vi "SIMPLE_Bulk_Stat.vi"() -> ()   [LabVIEW 2016]
uses:
  <vilib>/Instr/_visa.llb/VISA Set IO Buffer Mask.ctl
  <vilib>/Utility/miscctls.llb/LVPointTypeDef.ctl
  REV_2.lvlib
  <vilib>/Instr/_visa.llb/VISA Configure Serial Port (Instr).vi
  REV2_Stat_Addr.ctl
panel:
  out "Waveform Chart":dbl(graph)=240.78979051288226
  in  "Enum":enum16{"One_by_One", "Bulk"}(ring)
  in  "Stat_to_Read":T1[](array[typedef])=[8, 9] items=["Torque Enable", "Homing Complete", "Goal Id", "Goal Iq", "Goal Velo", "Goal Posi", "Present Id", "Present Iq", "Present Velo", "Present Posi", "Bus Voltage", "Temperature Winding", "Temperature MOSFET", "Temperature IC", "Error Status", "Iq_Temps"]
  in  "Data_to_Write":dbl[][](array[numeric])=[[0.0], [0.0], [0.0], [0.0], [0.0], [0.0], [0.0], [0.0], [0.0], [0.0], [0.0], [0.0]]
  in  "Stat_to_Write":T1[](array[typedef])=[3] items=["Torque Enable", "Homing Complete", "Goal Id", "Goal Iq", "Goal Velo", "Goal Posi", "Present Id", "Present Iq", "Present Velo", "Present Posi", "Bus Voltage", "Temperature Winding", "Temperature MOSFET", "Temperature IC", "Error Status", "Iq_Temps"]
  in  "IDs":u8[](array[numeric])=[1, 2, 3, 4, 5, 6, 7, 8, 9, 10, 11, 12]
  out "Data_2D":dbl[][](array[numeric])=[[-0.09640240669250488, 7372.0263671875], [-1.2603185176849365, -5385.19287109375], [-0.42314088344573975, 130929.453125], [-0.14840322732925415, 13840.2578125], [-0.6294983625411987, -4865.42578125], [0.10544928908348083, 128472.46875], [-1.5680679082870483, 28076.017578125], [-0.011024624109268188, -5347.7939453125], [1.180788278579712, 128403.328125], [-0.07580620050430298, 30035.9765625], [-0.3092707395553589, -5952.68359375], [-0.6351131200790405, 130700.546875]]
  in  "R/W":bool
  in  "Baud rate":u32=8000000
  in  "Com port":refnum<visa-resource-name>="COM7"
  in  "stop":bool
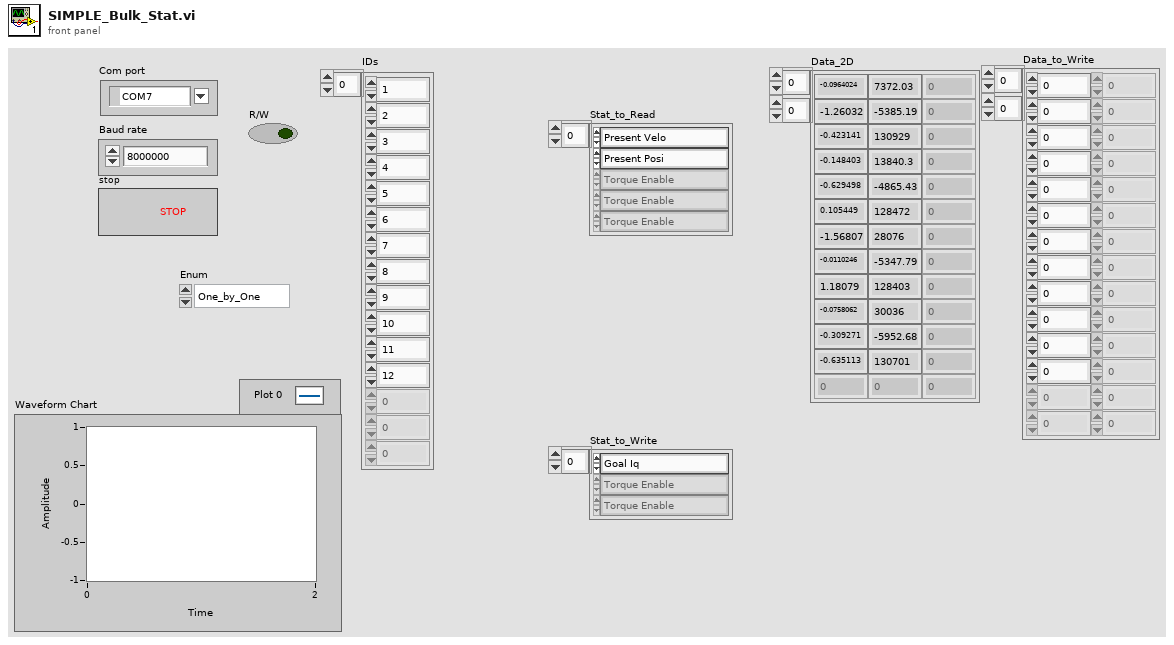
[diagram p1: front panel]
types:
  T1 = typedef "REV_2.lvlib/REV2_Stat_Addr.ctl" = u8
  T2 = typedef "LVPointTypeDef.ctl" = cluster{"Horizontal":i16, "Vertical":i16}
  T3 = typedef "VISA Set IO Buffer Mask.ctl" = u16
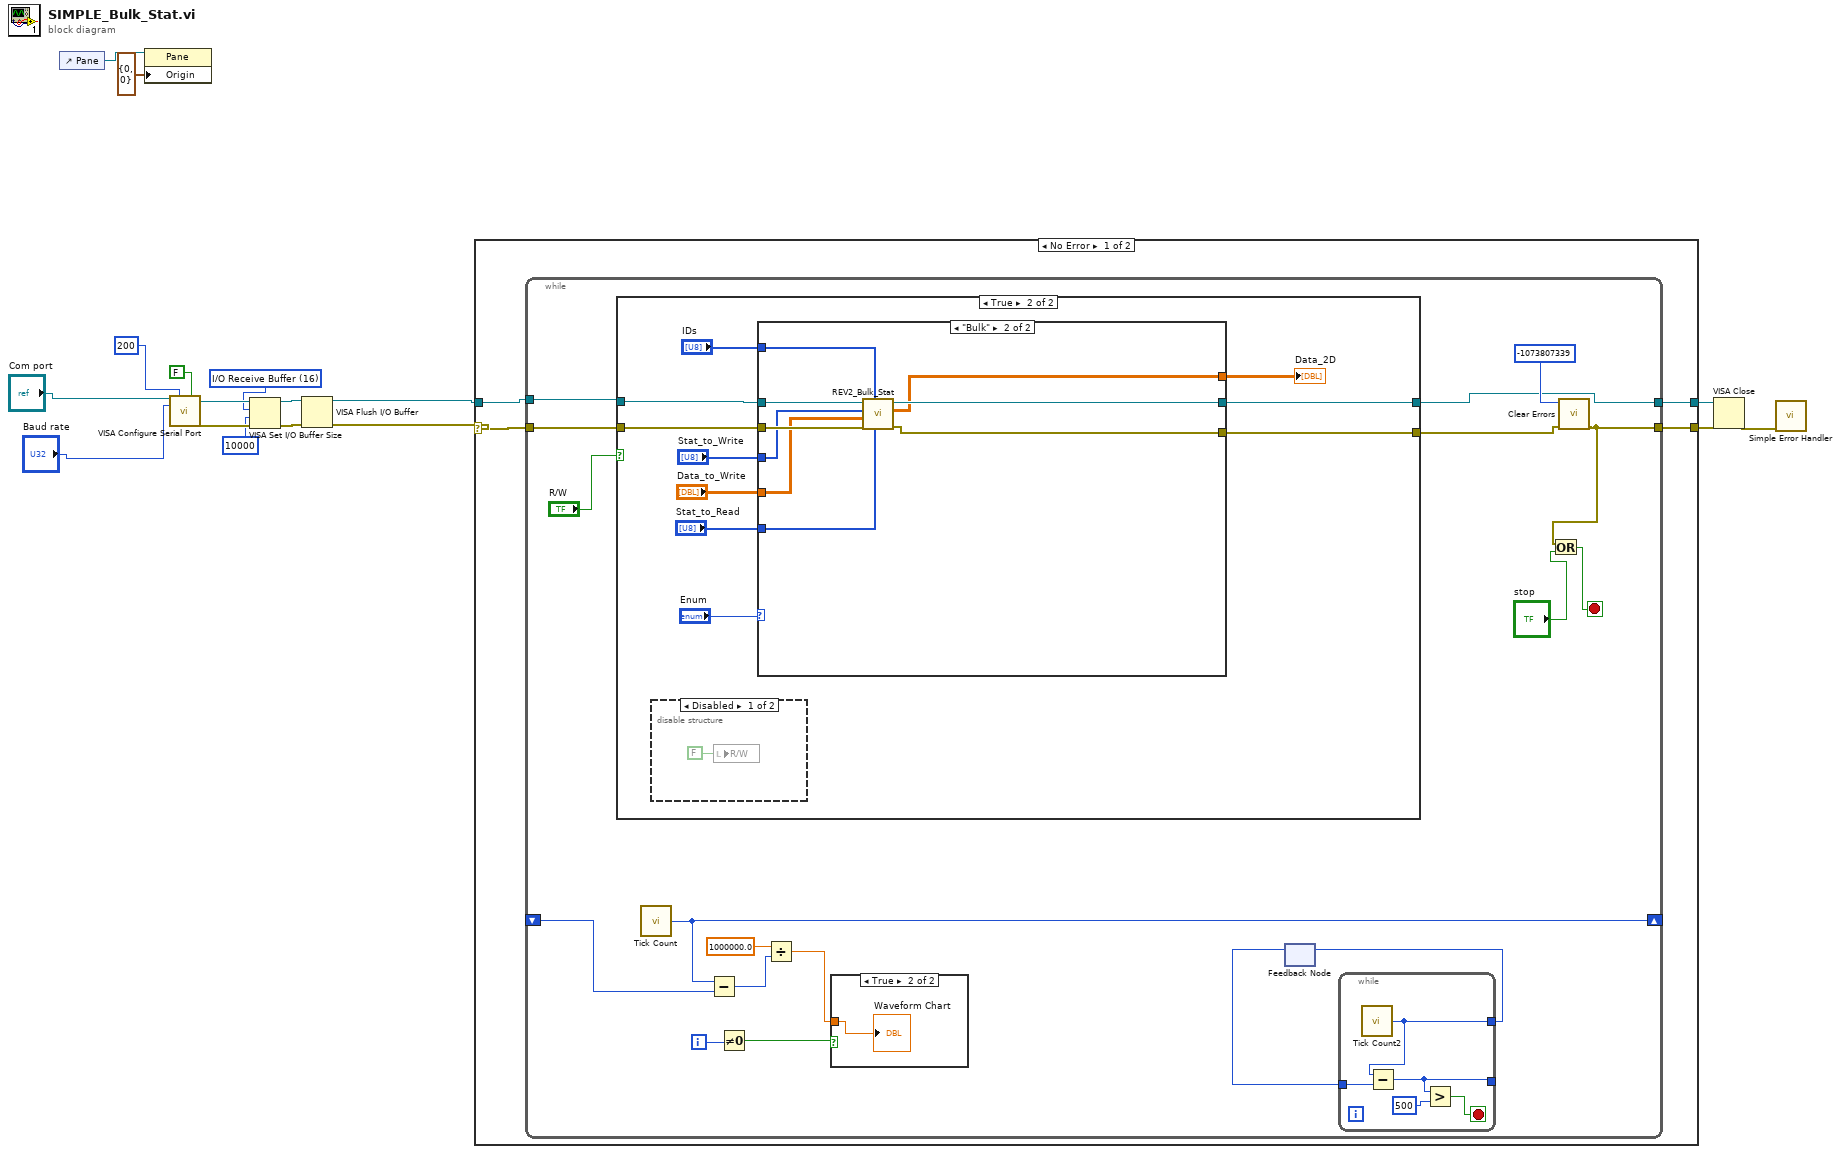
[diagram p0: block diagram]
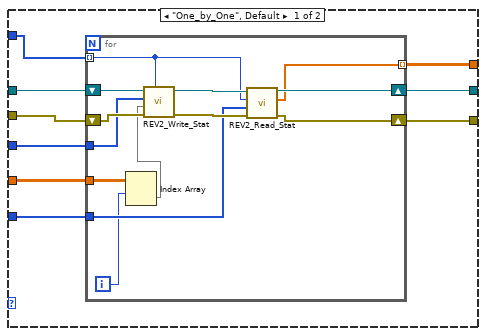
[diagram p5: hidden frame]
diagram:
  w9 = T3 16 items=["I/O Receive Buffer"=16, "I/O Transmit Buffer"=32, "I/O Receive and Transmit Buffer"=48] ("Mask")
  n1 = control-ref of="Pane"() -> (w4:refnum<vi>)
  n2 = property class="Pane"(reference=w4, "Origin"=T2 {"Horizontal"=0, "Vertical"=0}) -> ()  [unwired: 1 in, 2 out]
  n3 = call-poly "VISA Configure Serial Port"("VISA resource name"="Com port", "timeout (10sec)"=u32 200, "Enable Termination\nChar (T)"=FALSE ("Enable Termination\nChar (T)"), "baud rate (9600)"="Baud rate") -> ("VISA resource name out"=w10:refnum<visa-resource-name>, "error out"=w13:errorcluster)  [unwired: 10 in]
  n4 = VISA Set I/O Buffer Size(VISA resource name=w10, mask (16)=w9, size (4096)=u32 10000, error in (no error)=w13) -> (VISA resource name out=w11:refnum<visa-resource-name>, error out=w12:errorcluster)
  n5 = VISA Flush I/O Buffer(VISA resource name=w11, error in (no error)=w12) -> (VISA resource name out=w1:refnum<visa-resource-name>, error out=w2:errorcluster)  [unwired: 1 in]
  n6 = case shown="No Error" w2 {
    selector: w2 -> [w18 w90]
    tunnel: [w21 w90] -> w17
    tunnel: w1 -> [w20 w91]
    tunnel: [w19 w91] -> w15
    frame No Error {
      n7 = while {
        tunnel: w20 -> [w35]
        tunnel: w18 -> [w34]
        tunnel: [w31] -> w19
        tunnel: [w33] -> w21
        shift-right: [w30] -> _
        shift-left: _ -> [w29]
        i -> [w28]
        stop <- w38 stop-if-true
        n8 = case shown="True" "R/W" {
          tunnel: w34 -> [w47 w56]
          tunnel: w35 -> [w46 w57]
          tunnel: [w46 w54] -> w31
          tunnel: [w47 w55] -> w32
          frame False {
          }
          frame True {
            n9 = disable-structure shown="Disabled" {
              frame Disabled {
                n10 = local write "R/W"(FALSE ("write")) -> ()
              }
              frame Enabled {
              }
            }
            n11 = case shown="\"Bulk\"" "Enum" {
              tunnel: w57 -> [w66 w89]
              tunnel: w56 -> [w67 w88]
              tunnel: [w65 w87] -> w55
              tunnel: [w64 w86] -> w54
              tunnel: [w59 w85] -> w53
              tunnel: "IDs" -> [w63 w84]
              tunnel: "Stat_to_Write" -> [w62 w83]
              tunnel: "Data_to_Write" -> [w61 w82]
              tunnel: "Stat_to_Read" -> [w60 w81]
              frame "One_by_One", Default {
                n12 = for {
                  shift-right: [w76] -> w65
                  shift-left: w67 -> [w80]
                  shift-right: [w75] -> w64
                  shift-left: w66 -> [w79]
                  tunnel: w63 -> [w72] mode=indexing
                  tunnel: w62 -> [w74]
                  tunnel: w61 -> [w70]
                  tunnel: w60 -> [w73]
                  tunnel: [w71] -> w59 mode=indexing
                  i -> [w68]
                  n13 = Index Array(array=w70, index (row)=w68) -> (element=w69:dbl[])  [unwired: 1 in]
                  n14 = call "REV2_Write_Stat.vi"("ID"=w72, "error in (no error)"=w80, "Data"=w69, "Stat Addr"=w74, "VISA Refnum in"=w79) -> ("error out"=w77:errorcluster, "VISA Refnum out"=w78:refnum<visa-resource-name>)  [unwired: 5 in]
                  n15 = call "REV2_Read_Stat.vi"("error in (no error)"=w77, "Stat Address"=w73, "ID"=w72, "VISA Refnum in"=w78) -> ("error out"=w76:errorcluster, "Data"=w71:dbl[], "VISA Refnum out"=w75:refnum<visa-resource-name>)  [unwired: 4 in, 1 out]
                }
              }
              frame "Bulk" {
                n16 = call "REV2_Bulk_Stat.vi"("Stat_to_Read"=w81, "IDs"=w84, "error in (no error)"=w88, "Data_to_Write"=w82, "Stat_to_Write"=w83, "VISA Refnum in"=w89) -> ("error out"=w87:errorcluster, "Data_2D"=w85:dbl[][], "VISA Refnum out"=w86:refnum<visa-resource-name>)  [unwired: 3 in]
              }
            }
            "Data_2D" <- w53
          }
        }
        n17 = call "Tick Count"() -> ("Tick Count(uSec)"=w30:u32)
        n18 = Subtract(x=w30, y=w29) -> (x-y=w23:u32)
        n19 = Not Equal To 0?(x=w28) -> (x != 0?=w27:bool)
        n20 = Divide(x=1000000.0, y=w23) -> (x/y=w22:dbl)
        n21 = case shown="True" w27 {
          tunnel: w22 -> [_ w45]
          frame False {
          }
          frame True {
            "Waveform Chart" <- w45
          }
        }
        n22 = feedback #1() -> (w26:u32)  [unwired: 1 in]
        n23 = while {
          tunnel: w26 -> [w44]
          tunnel: [w43] -> w25
          tunnel: [w42] -> _
          stop <- w40 stop-if-true
          n24 = call "Tick Count2"() -> ("Tick Count(uSec)"=w43:u32)
          n25 = Subtract(x=w43, y=w44) -> (x-y=w42:u32)
          n26 = Greater?(x=w42, y=u32 500) -> (0:w40:bool)
        }
        n27 = feedback-in #1(w25) -> ()
        n28 = call <vilib>:"Clear Errors.vi"("error in (no error)"=w32, "specific error code to clear (0: all)"=-1073807339) -> ("error out"=w33:errorcluster)  [unwired: 4 in, 1 out]
        n29 = Or(x=w33, y="stop") -> (x .or. y?=w38:bool)
      }
    }
    frame Error {
    }
  }
  n30 = VISA Close(VISA resource name=w15, error in (no error)=w17) -> (error out=w7:errorcluster)
  n31 = call <vilib>:"Simple Error Handler.vi"("error in (no error)"=w7) -> ()  [unwired: 4 in, 5 out]
